vi "Read ESI Files on RT Target.vi"(8 "error in":errorcluster, 11 "Target IP":string) -> (0 "error out":errorcluster, 3 "Existing Target Profiles":string[](array[string]))   [LabVIEW 2019, in "SEECD System Explorer.lvlib"]
uses:
  SEECD System Explorer.lvlib
  <vilib>/FTP/NI_FTP.lvlib
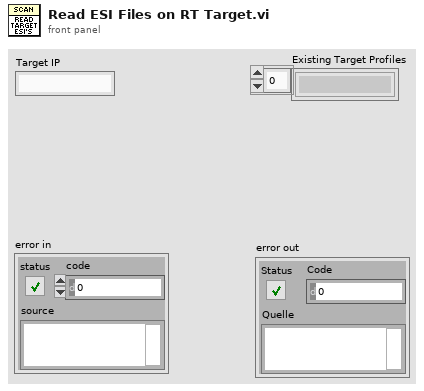
[diagram p1: front panel]
types:
  T1 = typedef "_fileTransferProtocol.ctl" = enum16{"Ftp", "WebDAV", "None"}
  T2 = typedef "_protocolSession.ctl" = cluster{"FTP session":T3, "WebDAV sssion":T4}
  T3 = typedef "NI_FTP.lvlib/FTP Session.ctl" = refnum<k5>
  T4 = typedef "NI_WebDAV.lvlib/SessionHandle.ctl" = refnum<k1>
  T5 = typedef "NI_FTP.lvlib/FTP File Info.ctl" = cluster{"type":enum16{"unknown", "file", "dir", "link"}, "permissions":string, "owner":string, "group":string, "size":i32, "date":string, "name":string, "link name":string}
  T6 = typedef "NI_WebDAV.lvlib/FileInfo.ctl" = cluster{"type":string, "size":u64, "last modification":timestamp, "display name":string, "uri":string}
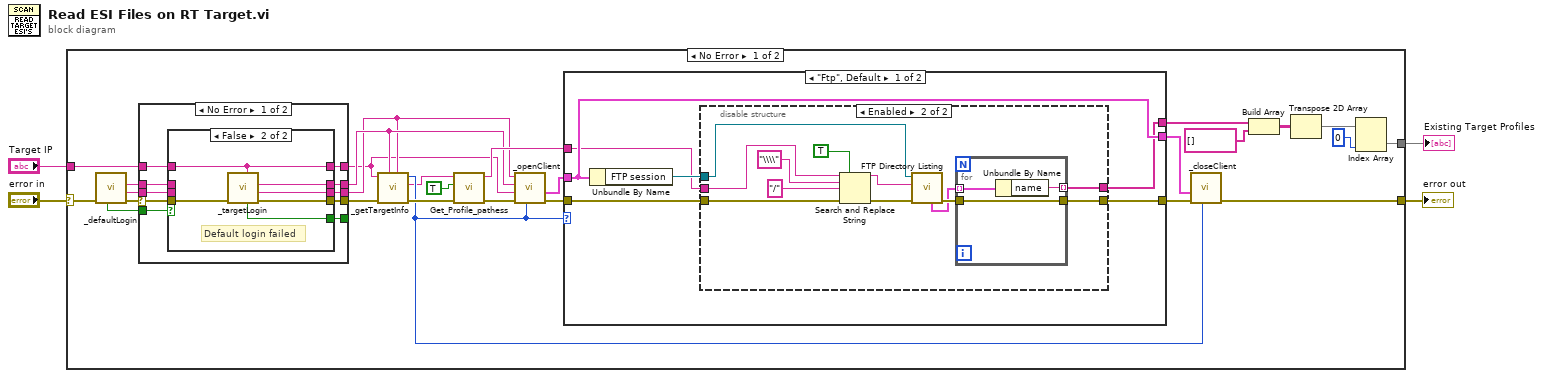
[diagram p0: block diagram]
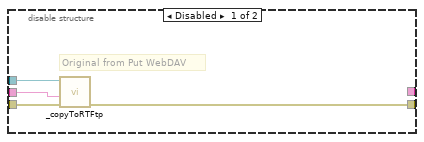
[diagram p4: hidden frame]
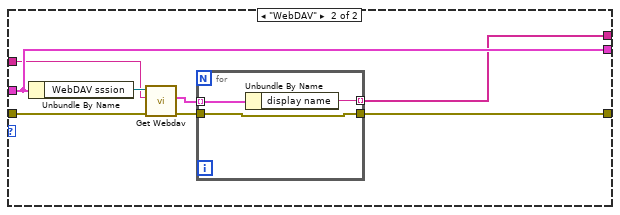
[diagram p5: hidden frame]
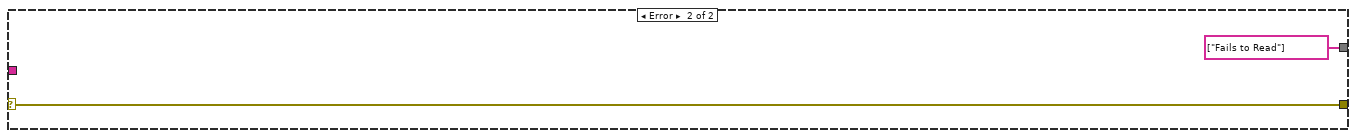
[diagram p6: hidden frame]
diagram:
  n1 = case shown="No Error" "error in" {
    selector: "error in" -> [w9 w90]
    tunnel: "Target IP" -> [w8 _]
    tunnel: [w28 w90] -> w2
    tunnel: [w27 string[] ["Fails to Read"]] -> w1
    frame No Error {
      n2 = call <resource>:"_defaultLogin.vi"("error in"=w9) -> ("error out"=w12:errorcluster, "password out"=w13:string, "user name out"=w14:string, "correct login?"=w11:bool)  [unwired: 7 in]
      n3 = case shown="No Error" w12 {
        selector: w12 -> [w35 w52]
        tunnel: [w41 _] -> w7
        tunnel: [w40 _] -> w6
        tunnel: [w39 _] -> _
        tunnel: [w38 w52] -> w10
        tunnel: w14 -> [w37 _]
        tunnel: w13 -> [w36 _]
        tunnel: w11 -> [w34 _]
        tunnel: w8 -> [w33 _]
        tunnel: [w32 _] -> w5
        frame No Error {
          n4 = case shown="False" w34 {
            tunnel: [w45 w51] -> w41
            tunnel: [w44 w50] -> w40
            tunnel: [w43 w49] -> w38
            tunnel: [_ w46] -> w39
            tunnel: w37 -> [w45 _]
            tunnel: w36 -> [w44 _]
            tunnel: w35 -> [w43 w48]
            tunnel: w33 -> [w42 w47]
            tunnel: [w42 w47] -> w32
            frame True {
            }
            frame False {
              # "Default login failed"
              n5 = call <resource>:"_targetLogin.vi"("Target IP"=w47, "error in"=w48) -> ("error out"=w49:errorcluster, "Password out"=w50:string, "Username out"=w51:string, "cancel?"=w46:bool)  [unwired: 6 in]
            }
          }
        }
        frame Error {
        }
      }
      n6 = call <resource>:"_getTargetInfo.vi"("password"=w6, "user name"=w7, "error in"=w10, "Target IP"=w5) -> ("error out"=w31:errorcluster, "Target OS"=w29:string, "protocol"=w30:T1)  [unwired: 4 in, 1 out]
      n7 = call "Get_Profile_pathess.vi"("error in (no error)"=w31, "Target?"=TRUE, "OSArch"=w29) -> ("error out"=w26:errorcluster, "profileDestPath"=w25:string)  [unwired: 7 in]
      n8 = call <resource>:"_openClient.vi"("protocol"=w30, "error in (no error)"=w26, "Target IP"=w5, "user name"=w7, "password"=w6) -> ("error out"=w15:errorcluster, "Cluster"=w18:T2)  [unwired: 5 in]
      n9 = case shown="\"Ftp\", Default" w30 {
        tunnel: w18 -> [w56 w83]
        tunnel: [w55 w80] -> w16
        tunnel: w15 -> [w58 w84]
        tunnel: [w56 w83] -> w17
        tunnel: w25 -> [w54 w82]
        tunnel: [w53 w78] -> w22
        frame "Ftp", Default {
          n10 = Unbundle By Name(w56) -> ("FTP session"=w57:T3)
          n11 = disable-structure shown="Enabled" {
            disable-tunnel: w58 -> [w62 w71]
            disable-tunnel: w57 -> [w61 w69]
            disable-tunnel: [w60 w66] -> w55
            disable-tunnel: w54 -> [w59 w72]
            disable-tunnel: [_ w65] -> w53
            frame Disabled {
              # "Original from Put WebDAV"
              n12 = call <resource>:"_copyToRTFtp.vi"("error in (no error)"=w62, "directory path"=w59, "TCP Network Connection in"=w61) -> ("error out"=w60:errorcluster)  [unwired: 7 in, 1 out]
            }
            frame Enabled {
              n13 = Search and Replace String(replace all?=TRUE ("replace all? (F)"), input string=w72, search string="\\\\", replace string="/" ("replace string (\"\")"), error in=w71) -> (result string=w68:string, error out=w70:errorcluster)  [unwired: 3 in, 2 out]
              n14 = call <vilib>:"FTP Directory Listing.vi"("error in (no error)"=w70, "directory path"=w68, "ftp session"=w69) -> ("error out"=w67:errorcluster, "dir list"=w64:T5[])  [unwired: 4 in, 3 out]
              n15 = for {
                tunnel: w67 -> [w77]
                tunnel: [w77] -> w66
                tunnel: w64 -> [w76] mode=indexing
                tunnel: [w75] -> w65 mode=indexing
                n16 = Unbundle By Name(w76) -> ("name"=w75:string)
              }
            }
          }
        }
        frame "WebDAV" {
          n17 = Unbundle By Name(w83) -> ("WebDAV sssion"=w85:T4)
          n18 = call "Get Webdav.vi"("error in (no error)"=w84, "relative uri"=w82, "Refnum in"=w85) -> ("error out"=w81:errorcluster, "file list"=w79:T6[])  [unwired: 6 in, 1 out]
          n19 = for {
            tunnel: w81 -> [w88]
            tunnel: [w88] -> w80
            tunnel: w79 -> [w87] mode=indexing
            tunnel: [w86] -> w78 mode=indexing
            n20 = Unbundle By Name(w87) -> ("display name"=w86:string)
          }
        }
      }
      n21 = call <resource>:"_closeClient.vi"("protocol"=w30, "error in"=w16, "session in"=w17) -> ("error out"=w28:errorcluster)  [unwired: 8 in]
      n22 = Build Array(w22, string[] [] ("Element")) -> (w24:string[][])
      n23 = Transpose 2D Array(2D array=w24) -> (transposed array=w21:string[][])
      n24 = Index Array(array=w21, index (col)=0) -> (element=w27:string[])  [unwired: 1 in]
    }
    frame Error {
    }
  }
  "error out" <- w2
  "Existing Target Profiles" <- w1
